vi "FPGA myRIOMain_v5.vi"() -> ()   [LabVIEW 2019]
doc: "Main FPGA VI\nUse the bitfile generated by this VI in the real-time code.\n\nv5: 16-pt Moving Average filter in AI sample loop"
uses:
  <vilib>/eio/EIONode/EIONode.xnode
  <vilib>/rvi/DataTransferAndStorage/Container/XNode/niFpgaContainer.xnode
  <vilib>/rvi/eio/common/nirviEmuTemplateMethod_errors.vi
  <vilib>/rvi/FIFO/Fifo_Resource/nirvififoEmulationRead.vi
  <vilib>/rvi/FIFO/Fifo_Resource/nirvififoEmulationWrite.vi
  FPGA functions/FPGA functions.lvlib
  <vilib>/rvi/FXPMathLib/FxpMul/XNode/nifxpmath_Multiplier.xnode
  <vilib>/rvi/FXPMathLib/sim/FxpSim.dll
  <vilib>/rvi/Analysis/measure/butterworth/XNode/niFpgaButterworthFilter.xnode
  <vilib>/rvi/DataTransferAndStorage/Register/Emulation/niFpgaRegisterEmulation.vi
  TypeDefs/AO mode TabCtrl.ctl
  TypeDefs/SamplingModeEnum.ctl
panel:
  in  "AI Process Time [ticks]":u32=120
  out "Sample Freq. \ntoo high?":bool
  out "Processing Loop time [ticks]":u32
  out "AI Process. Freq.\ntoo high?":bool
  in  "Scaled Butterworth Coeffs":i32[](array[numeric])=[-1036986264, 2110353124, 93741, -1058362983, 2131726043, 94691]
  in  "Sampling Mode":T1
  in  "AO mode":T2
  in  "AO Out [V]":fxp<+/-,18,5> format="%#.6g"
  in  "AO enable?":bool
  out "AI In [V]":fxp<+/-,25,5> format="%#.6g"
  out "FPGA AO DMA\nOverflow?":bool
  out "Int. Output":i16
  out "Raw Int. Input":fxp<+/-,16,12> format="%.8g"
  in  "Sample Time [ticks]":u32=120
  out "AO Loop time [ticks]":u32
  out "AI Loop time [ticks]":u32
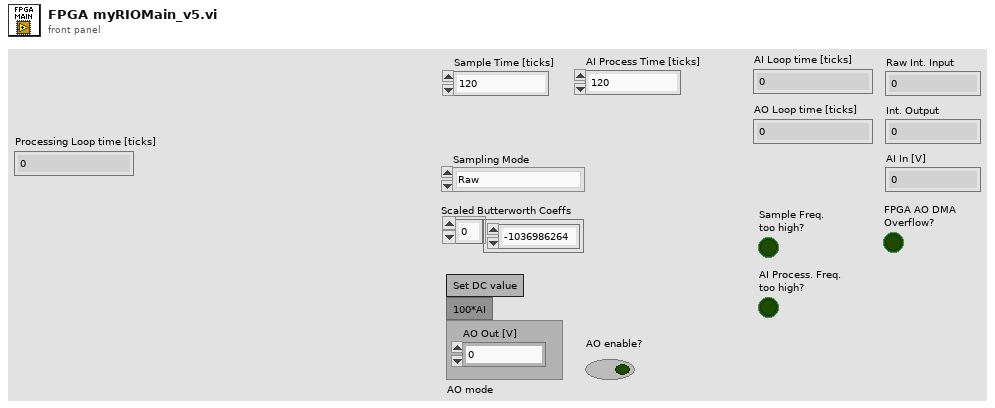
[diagram p1: front panel]
types:
  T1 = typedef "SamplingModeEnum.ctl" = enum16{"Raw", "4pt MA (AI)", "LPF (Proc.)", "4pt MA (AI) + LPF (Proc.)", "4pt MA (Proc.) + LPF (Proc.)"}
  T2 = typedef "AO mode TabCtrl.ctl" = enum32{"Set DC value", "100*AI"}
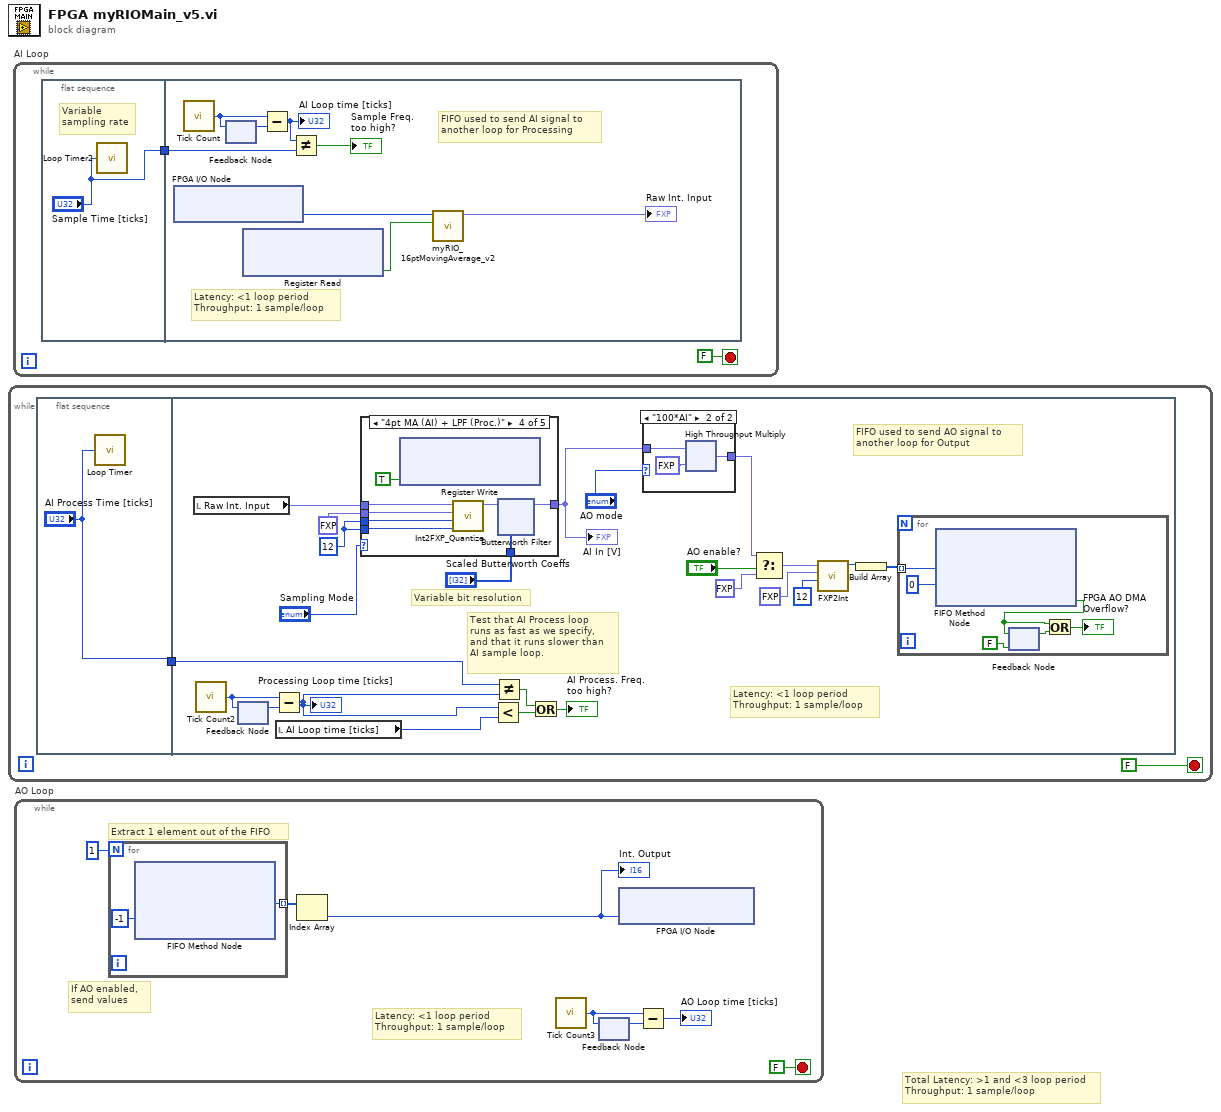
[diagram p0: block diagram]
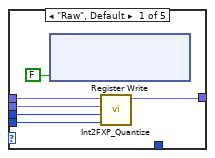
[diagram p2: hidden frame]
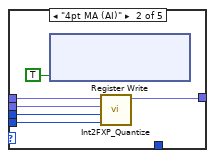
[diagram p3: hidden frame]
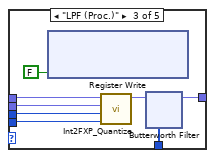
[diagram p4: hidden frame]
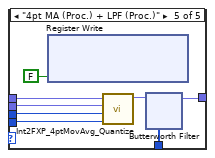
[diagram p5: hidden frame]
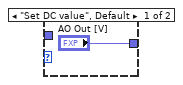
[diagram p6: hidden frame]
diagram:
  # "Total Latency: >1 and <3 loop period\nThroughput: 1 sample/loop"
  n1 = while {
    stop <- FALSE stop-if-true
    n2 = flat-sequence {
      tunnel: ["AI Process Time [ticks]"] -> w1
      tunnel: w1 -> [w6]
      frame #0 {
        n3 = call "Loop Timer"("Count(Ticks)"="AI Process Time [ticks]") -> ()  [unwired: 1 out]
      }
      frame #1 {
        w4 = i8 12 ("Input Bit resolution")
        # "Test that AI Process loop\nruns as fast as we specify,\nand that it runs slower than \nAI sample loop."
        # "Variable bit resolution"
        # "Latency: <1 loop period\nThroughput: 1 sample/loop"
        # "FIFO used to send AO signal to \nanother loop for Output"
        n4 = local read "Raw Int. Input"() -> (w11:fxp<+/-,16,12>)
        n5 = call "Tick Count2"() -> ("Tick Count(Ticks)"=w13:u32)
        n6 = feedback #1() -> (w12:u32)  [unwired: 1 in]
        n7 = feedback-in #1(w13) -> ()
        n8 = Subtract(x=w13, y=w12) -> (x-y=w5:u32)
        "Processing Loop time [ticks]" <- w5
        n9 = local read "AI Loop time [ticks]"() -> (w10:u32)
        n10 = case shown="\"4pt MA (AI) + LPF (Proc.)\"" "Sampling Mode" {
          tunnel: w4 -> [w32 w38 w43 w59 w77]
          tunnel: fxp<+,8,4> 10.0 ("Multiplier") -> [w31 w37 w44 w60 w78]
          tunnel: w4 -> [w30 w36 w42 w58 w76]
          tunnel: "Scaled Butterworth Coeffs" -> [_ _ w45 w61 w74]
          tunnel: [w29 w35 w41 w57 w73] -> w14
          tunnel: w11 -> [w28 w34 w40 w56 w72]
          frame "Raw", Default {
            n11 = xnode ("Register Write")("Data"=FALSE) -> ()  [unwired: 1 in, 1 out]
            n12 = call "Int2FXP_Quantize.vi"("Output Bit resolution"=w30, "Input Bit resolution"=w32, "Multiplier"=w31, "Input (Int)"=w28) -> ("Output (FXP)"=w29:fxp<+/-,25,5>)  [unwired: 7 in]
          }
          frame "4pt MA (AI)" {
            n13 = xnode ("Register Write")("Data"=TRUE) -> ()  [unwired: 1 in, 1 out]
            n14 = call "Int2FXP_Quantize.vi"("Output Bit resolution"=w36, "Input Bit resolution"=w38, "Multiplier"=w37, "Input (Int)"=w34) -> ("Output (FXP)"=w35:fxp<+/-,25,5>)  [unwired: 7 in]
          }
          frame "LPF (Proc.)" {
            n15 = xnode ("Register Write")("Data"=FALSE) -> ()  [unwired: 1 in, 1 out]
            n16 = call "Int2FXP_Quantize.vi"("Output Bit resolution"=w42, "Input Bit resolution"=w43, "Multiplier"=w44, "Input (Int)"=w40) -> ("Output (FXP)"=w46:fxp<+/-,25,5>)  [unwired: 7 in]
            n17 = xnode "Butterworth Filter"("input data"=w46, "scaled coefficients"=w45) -> ("output data"=w41:fxp<+/-,25,5>)  [unwired: 1 in]
          }
          frame "4pt MA (AI) + LPF (Proc.)" {
            n18 = xnode ("Register Write")("Data"=TRUE) -> ()  [unwired: 1 in, 1 out]
            n19 = call "Int2FXP_Quantize.vi"("Output Bit resolution"=w58, "Input Bit resolution"=w59, "Multiplier"=w60, "Input (Int)"=w56) -> ("Output (FXP)"=w62:fxp<+/-,25,5>)  [unwired: 7 in]
            n20 = xnode "Butterworth Filter"("input data"=w62, "scaled coefficients"=w61) -> ("output data"=w57:fxp<+/-,25,5>)  [unwired: 1 in]
          }
          frame "4pt MA (Proc.) + LPF (Proc.)" {
            n21 = xnode ("Register Write")("Data"=FALSE) -> ()  [unwired: 1 in, 1 out]
            n22 = call "Int2FXP_4ptMovAvg_Quantize.vi"("Output Bit resolution"=w76, "Input Bit resolution"=w77, "Multiplier"=w78, "Input (Int)"=w72) -> ("Output (FXP)"=w75:fxp<+/-,25,5>)  [unwired: 7 in]
            n23 = xnode "Butterworth Filter"("input data"=w75, "scaled coefficients"=w74) -> ("output data"=w73:fxp<+/-,25,5>)  [unwired: 1 in]
          }
        }
        "AI In [V]" <- w14
        n24 = Less?(x=w5, y=w10) -> (x < y?=w7:bool)
        n25 = Not Equal?(x=w6, y=w5) -> (x != y?=w8:bool)
        n26 = Or(x=w8, y=w7) -> (x .or. y?=→"AI Process. Freq.\ntoo high?":bool)
        n27 = case shown="\"100*AI\"" "AO mode" {
          tunnel: ["AO Out [V]" w88] -> w19
          tunnel: w14 -> [_ w90]
          frame "Set DC value", Default {
          }
          frame "100*AI" {
            n28 = xnode ("High Throughput Multiply")("x"=w90, "y"=fxp<+,5,7> 100.0) -> ("x*y"=w88:fxp<+/-,18,5>)
          }
        }
        n29 = Select(t=w19, s="AO enable?", f=fxp<+/-,18,5> 0.0) -> (s? t:f=w20:fxp<+/-,18,5>)
        n30 = call "FXP2Int.vi"("Output Bit resolution"=i8 12 ("Bit resolution"), "Multiplier"=fxp<+,18,-1> 0.10000038146972656, "Input (FXP)"=w20) -> ("Output (Int)"=w26:i16)  [unwired: 8 in]
        n31 = Build Array(w26) -> (w21:i16[])
        n32 = for {
          tunnel: w21 -> [w93] mode=indexing
          n33 = xnode ("FIFO Method Node")("Element"=w93, "Timeout"=0) -> ("Timed Out?"=w91:bool)  [unwired: 1 in, 1 out]
          n34 = feedback-in #2(w91) -> ()
          n35 = feedback #2(FALSE ("Timed Out?")) -> (w95:bool)
          n36 = Or(x=w91, y=w95) -> (x .or. y?=→"FPGA AO DMA\nOverflow?":bool)
        }
      }
    }
  }
  n37 = while "AI Loop" {
    stop <- FALSE stop-if-true
    n38 = flat-sequence {
      tunnel: ["Sample Time [ticks]"] -> w97
      tunnel: w97 -> [w104]
      frame #0 {
        # "Variable\nsampling rate"
        n39 = call "Loop Timer2"("Count(Ticks)"="Sample Time [ticks]") -> ()  [unwired: 1 out]
      }
      frame #1 {
        # "FIFO used to send AI signal to \nanother loop for Processing"
        # "Latency: <1 loop period\nThroughput: 1 sample/loop"
        n40 = xnode "FPGA I/O Node"() -> ("ConnectorC/AI0"=w102:i16)  [unwired: 1 in, 1 out]
        n41 = call "Tick Count"() -> ("Tick Count(Ticks)"=w107:u32)
        n42 = feedback #3() -> (w106:u32)  [unwired: 1 in]
        n43 = feedback-in #3(w107) -> ()
        n44 = xnode ("Register Read")() -> ("Data"=w100:bool)  [unwired: 1 in, 1 out]
        n45 = Subtract(x=w107, y=w106) -> (x-y=w105:u32)
        "AI Loop time [ticks]" <- w105
        n46 = Not Equal?(x=w105, y=w104) -> (x != y?=→"Sample Freq. \ntoo high?":bool)
        n47 = call "myRIO_16ptMovingAverage_v2.vi"("Enable?"=w100, "Raw input"=w102) -> ("Avg. output"=→"Raw Int. Input":fxp<+/-,16,12>)  [unwired: 9 in]
      }
    }
  }
  n48 = while "AO Loop" {
    stop <- FALSE stop-if-true
    # "Latency: <1 loop period\nThroughput: 1 sample/loop"
    # "If AO enabled, \nsend values"
    # "Extract 1 element out of the FIFO"
    n49 = for {
      N: 1 -> [_]
      tunnel: [w116] -> w110 mode=indexing
      n50 = xnode ("FIFO Method Node")("Timeout"=-1) -> ("Element"=w116:i16)  [unwired: 1 in, 2 out]
    }
    n51 = Index Array(array=w110) -> (element=w108:i16)  [unwired: 1 in]
    "Int. Output" <- w108
    n52 = call "Tick Count3"() -> ("Tick Count(Ticks)"=w113:u32)
    n53 = feedback #4() -> (w112:u32)  [unwired: 1 in]
    n54 = feedback-in #4(w113) -> ()
    n55 = xnode "FPGA I/O Node"("ConnectorC/AO0"=w108) -> ()  [unwired: 1 in, 1 out]
    n56 = Subtract(x=w113, y=w112) -> (x-y=→"AO Loop time [ticks]":u32)
  }
